vi "Get Object ACL.vi"(6 "Version ID":string, 8 "error in (no error)":errorcluster, 9 "Bucket":string, 10 "Path":string) -> (0 "error out":errorcluster, 3 "AccessControlPolicy":T1)   [LabVIEW 2011, in "LV Interface for Amazon S3.lvlib"]
doc: "This operation <B>returns the access control list (ACL)</B> of an object. To use this operation, <B>you must have READ_ACP access</B> to the object."
uses:
  LV Interface for Amazon S3.lvlib
  Typedefs/AMZ_S3_API_AccessControlPolicy.ctl
  Typedefs/AMZ_S3_API_Owner.ctl
  Typedefs/AMZ_S3_API_Bucket ACL Permission.ctl
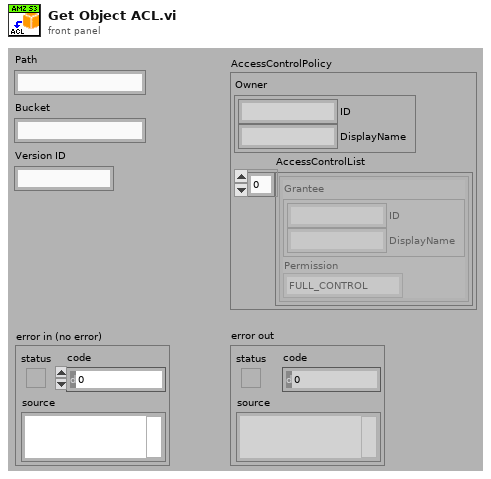
[diagram p1: front panel]
types:
  T1 = typedef "LV Interface for Amazon S3.lvlib/AMZ_S3_API_AccessControlPolicy.ctl" = cluster{"Owner":T2, "AccessControlList":cluster{"Grantee":T2, "Permission":T3}[]}
  T2 = typedef "LV Interface for Amazon S3.lvlib/AMZ_S3_API_Owner.ctl" = cluster{"ID":string, "DisplayName":string}
  T3 = typedef "LV Interface for Amazon S3.lvlib/AMZ_S3_API_Bucket ACL Permission.ctl" = enum16{"FULL_CONTROL", "WRITE", "WRITE_ACP", "READ", "READ_ACP"}
  T4 = typedef "LV Interface for Amazon S3.lvlib/AMZ_S3_Call Results.ctl" = enum16{"Success", "UndefinedError", "AccessDenied", "AccountProblem", "AmbiguousGrantByEmailAddress", "BadDigest", "BucketAlreadyExists", "BucketAlreadyOwnedByYou", "BucketNotEmpty", "CredentialsNotSupported", "CrossLocationLoggingProhibited", "EntityTooSmall", "EntityTooLarge", "ExpiredToken", "IllegalVersioningConfigurationException", "IncompleteBody", "IncorrectNumberOfFilesInPostRequest", "InlineDataTooLarge", "InternalError", "InvalidAccessKeyId", "InvalidAddressingHeader", "InvalidArgument", "InvalidBucketName", "InvalidDigest", "InvalidLocationConstraint", "InvalidPart", "InvalidPartOrder", "InvalidPayer", "InvalidPolicyDocument", "InvalidRange", "InvalidSecurity", "InvalidSOAPRequest", "InvalidStorageClass", "InvalidTargetBucketForLogging", "InvalidToken", "InvalidURI", "KeyTooLong", "MalformedACLError", "MalformedPOSTRequest", "MalformedXML", "MaxMessageLengthExceeded", "MaxPostPreDataLengthExceededError", "MetadataTooLarge", "MethodNotAllowed", "MissingAttachment", "MissingContentLength", "MissingRequestBodyError", "MissingSecurityElement", "MissingSecurityHeader", "NoLoggingStatusForKey", "NoSuchBucket", "NoSuchKey", "NoSuchUpload", "NoSuchVersion", "NotImplemented", "NotSignedUp", "OperationAborted", "PermanentRedirect", "PreconditionFailed", "Redirect", "RequestIsNotMultiPartContent", "RequestTimeout", "RequestTimeTooSkewed", "RequestTorrentOfBucketError", "SignatureDoesNotMatch", "SlowDown", "TemporaryRedirect", "TokenRefreshRequired", "TooManyBuckets", "UnexpectedContent", "UnresolvableGrantByEmailAddress", "UserKeyMustBeSpecified", "LabVIEWError"}
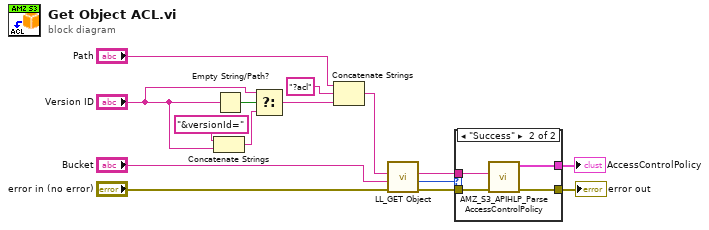
[diagram p0: block diagram]
diagram:
  n1 = Concatenate Strings("&versionId=", "Version ID") -> (w10:string)
  n2 = Empty String/Path?(string/path="Version ID") -> (empty?=w13:bool)
  n3 = Select(t="Version ID", s=w13, f=w10) -> (s? t:f=w9:string)
  n4 = Concatenate Strings("Path", "?acl" ("string"), w9) -> (w6:string)
  n5 = call "LL_GET Object.vi"("error in (no error)"="error in (no error)", "Bucket"="Bucket", "Path and query string"=w6) -> ("error out"=w5:errorcluster, "Call Result"=w4:T4, "Response body"=w3:string)  [unwired: 5 in, 1 out]
  n6 = case shown="\"Success\"" w4 {
    tunnel: w5 -> [w16 w20]
    tunnel: w3 -> [_ w19]
    tunnel: [w16 w18] -> w1
    tunnel: [_ w17] -> w2
    frame Default {
    }
    frame "Success" {
      n7 = call "AMZ_S3_APIHLP_Parse AccessControlPolicy.vi"("error in (no error)"=w20, "Response body"=w19) -> ("error out"=w18:errorcluster, "AccessControlPolicy"=w17:T1)  [unwired: 8 in]
    }
  }
  "AccessControlPolicy" <- w2
  "error out" <- w1
